vi "ELL9_Switching_with_Failed_Move_Correction.vi"() -> ()   [LabVIEW 2017]
uses:
  U:/UDocuments/Thorlabs.Elliptec.ELLO_DLL.dll
  Thorlabs.Elliptec.ELLO_DLL.dll
panel:
  in  "Stop VI":bool
  in  "COM Port":string="COM5"
  in  "Device Address":string="0"
  in  "Position 2":bool
  in  "Position 1":bool caption="Home"
  in  "Position 3":bool
  in  "Position 4":bool
  in  "Home":bool
  # "Notes:"
  # "This VI is only designed for use with the ELL9 stages.They can be running \"Daisy-Chained\" or through the ELLB Control Bus Distributor \nThe stages can not share the same address\n\nIf, when running the VI for the first time, you get a popup as illustrated below, then click Browse and navigate to the \nThorlabs.Elliptec.ELLO_DLL.dll file in the ELLO software installation directory. This can be copied to the folder you are \nrunning the VI from."
  # "Thorlabs Hardware: ELL9 - Four-Position Slider: SM1 Threads, 30 mm Cage Compatible\nhttps://www.thorlabs.com/thorproduct.cfm?partnumber=ELL9\n\nDescription: This VI will enable you to communicate with two ELL9 filter mounts. It covers connecting to the relevant COM port and addressing the desired device as well as homing the device and moving between the 16  filter positions using a case structure and while loop. \n\nIt is assumed  that you know the device address of your stage. By default this will be 0 unless changed by a user. It can be any value in Hex from 0 to F. If the device address is unknown then this is most easily found through the ELLO software: \nhttps://www.thorlabs.com/software_pages/ViewSoftwarePage.cfm?Code=ELL"
  # "Instructions:"
  # "1) Connect your devices to the USB Interface board via the ribbon cable. \n2) Connect power to the board and wait for approximately 15 seconds. As soon as the stage has power it will attempt a frequency search.\n     If the power is insufficient the board will not find the correct operating frequencies. This is why the USB is attached last. Ensure   \n     sufficient current is supplied for the number of attached stages.\n3) Connect the interface board to the PC via the USB cable.\n4) Enter the addresses of the stage you are using and the COM port you are communicating with the USB over.\n5) Run the VI.\n6) Select the position you want and allow the move to complete before choosing another."
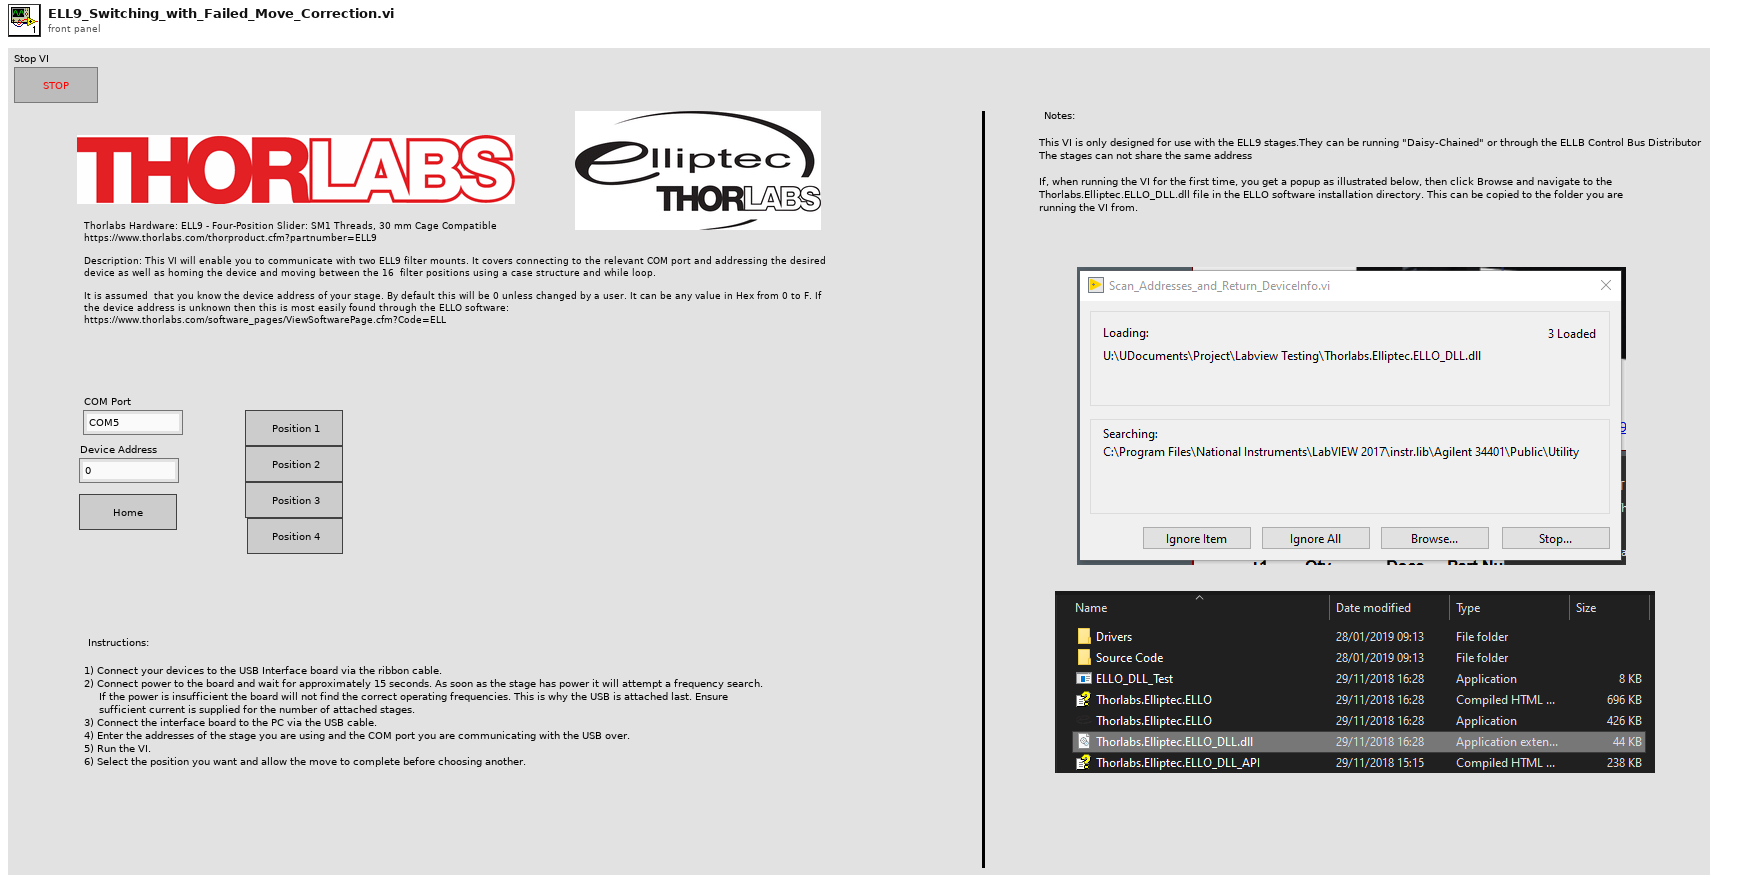
[diagram p1: front panel]
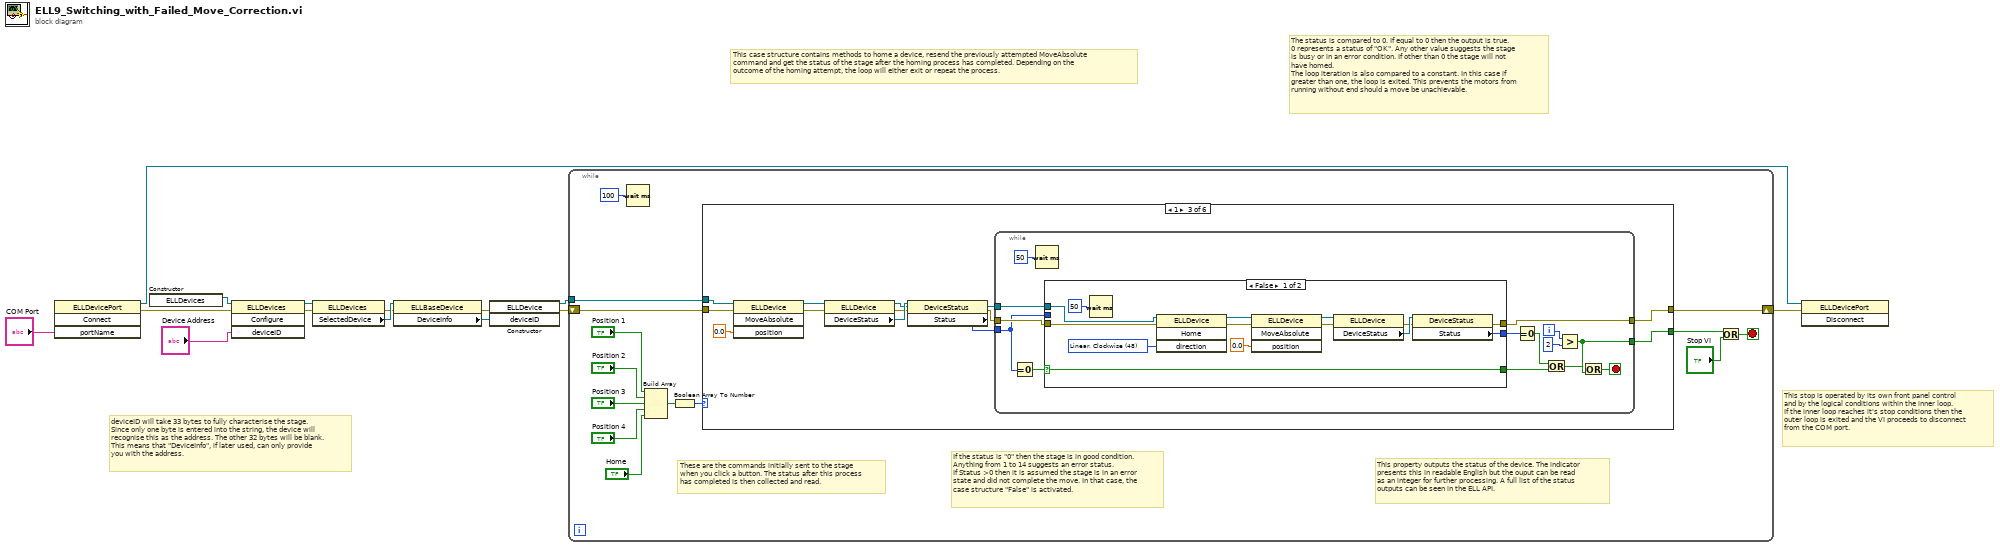
[diagram p0: block diagram]
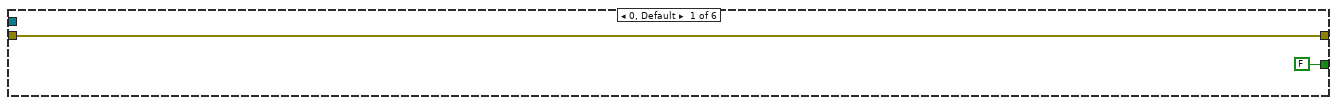
[diagram p2: hidden frame]
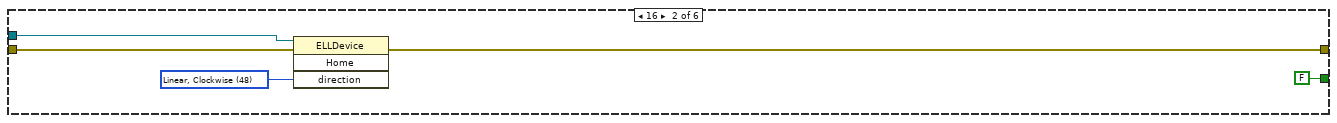
[diagram p3: hidden frame]
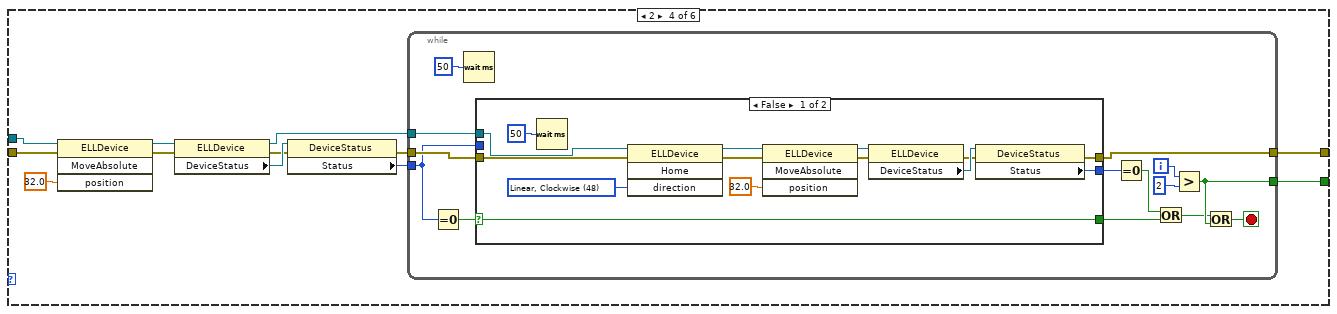
[diagram p5: hidden frame]
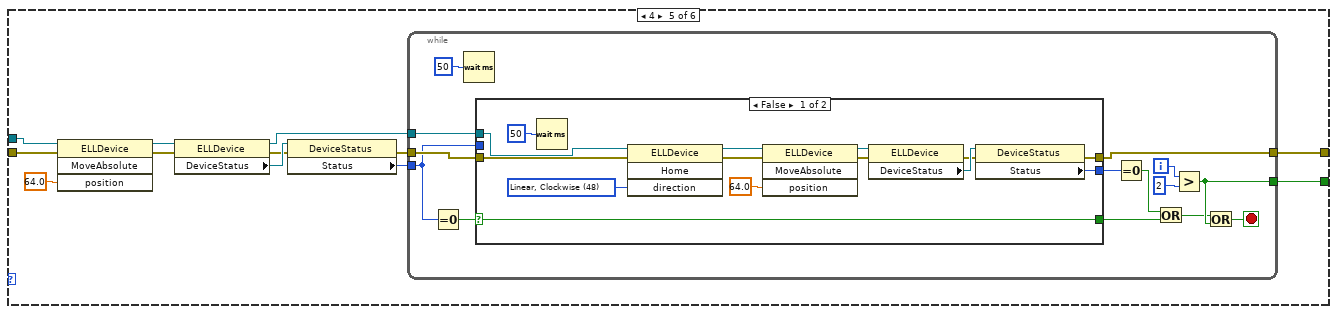
[diagram p7: hidden frame]
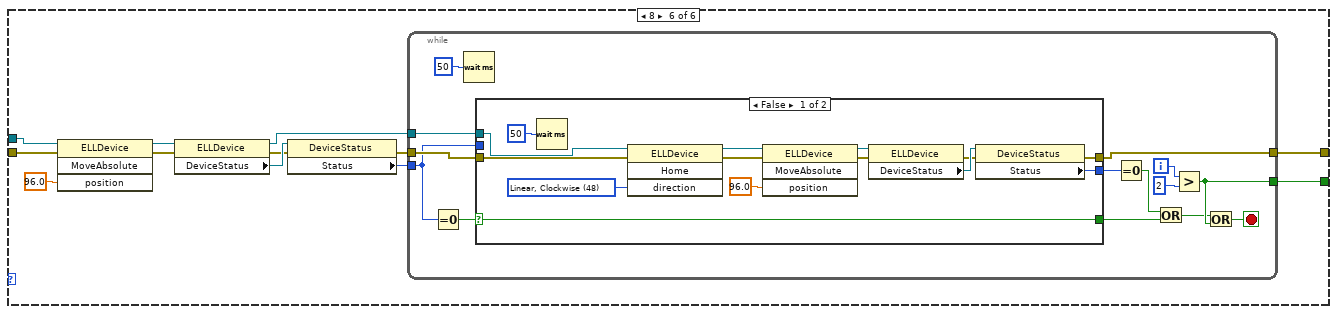
[diagram p9: hidden frame]
diagram:
  # "This case structure contains methods to home a device, resend the previously attempted MoveAbsolute \ncommand and get the status of the stage after the homing process has completed. Depending on the \noutcome of the homing attempt, the loop will either exit or repeat the process."
  # "This stop is operated by its own front panel control\nand by the logical conditions within the inner loop.\nIf the inner loop reaches it's stop conditions then the\nouter loop is exited and the VI proceeds to disconnect\nfrom the COM port."
  # "The status is compared to 0. If equal to 0 then the output is true.\n0 represents a status of \"OK\". Any other value suggests the stage\nis busy or in an error condition. If other than 0 the stage will not\nhave homed.\nThe loop iteration is also compared to a constant. In this case if\ngreater than one, the loop is exited. This prevents the motors from\nrunning without end should a move be unachievable."
  # "deviceID will take 33 bytes to fully characterise the stage. \nSince only one byte is entered into the string, the device will \nrecognise this as the address. The other 32 bytes will be blank.\nThis means that \"DeviceInfo\", if later used, can only provide \nyou with the address."
  n1 = invoke class="ELLDevicePort" method="Connect"("portName"="COM Port") -> (reference out=w14:refnum<k24>, error out=w2:errorcluster)  [unwired: 3 in, 2 out]
  n2 = constructor class="ELLDevices"() -> (reference out=w3:refnum<k24>)  [unwired: 3 in, 2 out]
  n3 = invoke class="ELLDevices" method="Configure"(reference=w3, error in=w2, "deviceID"="Device Address") -> (reference out=w11:refnum<k24>, error out=w10:errorcluster)  [unwired: 1 in, 2 out]
  n4 = property class="ELLDevices"(reference=w11, error in=w10) -> (error out=w6:errorcluster, "SelectedDevice"=w7:refnum<k24>)  [unwired: 1 out]
  n5 = property class="ELLBaseDevice"(reference=w7, error in=w6) -> (error out=w8:errorcluster, "DeviceInfo"=w9:refnum<k24>)  [unwired: 1 out]
  n6 = constructor class="ELLDevice"(error in=w8, "deviceID"=w9) -> (reference out=w5:refnum<k24>, error out=w4:errorcluster)  [unwired: 2 in, 2 out]
  n7 = while {
    shift-right: [w15] -> w13
    shift-left: w4 -> [w21]
    tunnel: w5 -> [w19]
    stop <- w18 stop-if-true
    # "These are the commands initially sent to the stage\nwhen you click a button. The status after this process\nhas completed is then collected and read."
    # "This property outputs the status of the device. The indicator\npresents this in readable English but the ouput can be read\nas an integer for further processing. A full list of the status \noutputs can be seen in the ELL API."
    # "If the status is \"0\" then the stage is in good condition.\nAnything from 1 to 14 suggests an error status. \nIf Status >0 then it is assumed the stage is in an error \nstate and did not complete the move. In that case, the\ncase structure \"False\" is activated."
    n8 = Wait (ms)(milliseconds to wait=u32 100) -> ()  [unwired: 1 out]
    n9 = Build Array("Position 1", "Position 2", "Position 3", "Position 4", "Home") -> (w28:bool[])
    n10 = Boolean Array To Number(Boolean array=w28) -> (number=w24:u32)
    n11 = case shown="1" w24 {
      tunnel: w21 -> [w30 w34 w46 w89 w132 w175]
      tunnel: w19 -> [_ w33 w45 w88 w131 w174]
      tunnel: [w30 w32 w40 w83 w126 w169] -> w15
      tunnel: [FALSE FALSE w36 w79 w122 w165] -> w17
      frame 0, Default {
      }
      frame 16 {
        w35 = 48 items=["Linear, Clockwise"=48, "AntiClockwise"=49] ("direction")
        n12 = invoke class="ELLDevice" method="Home"(reference=w33, error in=w34, "direction"=w35) -> (error out=w32:errorcluster)  [unwired: 1 in, 3 out]
      }
      frame 1 {
        n13 = invoke class="ELLDevice" method="MoveAbsolute"(reference=w45, error in=w46, "position"=0.0) -> (reference out=w42:refnum<k24>, error out=w41:errorcluster)  [unwired: 1 in, 2 out]
        n14 = property class="ELLDevice"(reference=w42, error in=w41) -> (reference out=w37:refnum<k24>, error out=w43:errorcluster, "DeviceStatus"=w44:refnum<k24>)
        n15 = property class="DeviceStatus"(reference=w44, error in=w43) -> (error out=w39:errorcluster, "Status"=w38:i32)  [unwired: 1 out]
        n16 = while {
          tunnel: [w58] -> w36
          tunnel: w37 -> [w51]
          tunnel: w38 -> [w48]
          tunnel: w39 -> [w49]
          tunnel: [w50] -> w40
          i -> [w61]
          stop <- w59 stop-if-true
          n17 = Equal To 0?(x=w48) -> (x = 0?=w53:bool)
          n18 = Wait (ms)(milliseconds to wait=u32 50) -> ()  [unwired: 1 out]
          n19 = case shown="False" w53 {
            selector: w53 -> [w62 w78]
            tunnel: w49 -> [w65 w77]
            tunnel: [w71 w76] -> w57
            tunnel: [w62 w78] -> w54
            tunnel: w51 -> [w67 _]
            tunnel: [w66 w77] -> w50
            tunnel: w48 -> [_ w76]
            frame False {
              w72 = 48 items=["Linear, Clockwise"=48, "AntiClockwise"=49] ("direction")
              n20 = Wait (ms)(milliseconds to wait=u32 50) -> ()  [unwired: 1 out]
              n21 = invoke class="ELLDevice" method="Home"(reference=w67, error in=w65, "direction"=w72) -> (reference out=w73:refnum<k24>, error out=w74:errorcluster)  [unwired: 1 in, 2 out]
              n22 = invoke class="ELLDevice" method="MoveAbsolute"(reference=w73, error in=w74, "position"=0.0) -> (reference out=w64:refnum<k24>, error out=w63:errorcluster)  [unwired: 1 in, 2 out]
              n23 = property class="ELLDevice"(reference=w64, error in=w63) -> (error out=w69:errorcluster, "DeviceStatus"=w70:refnum<k24>)  [unwired: 1 out]
              n24 = property class="DeviceStatus"(reference=w70, error in=w69) -> (error out=w66:errorcluster, "Status"=w71:i32)  [unwired: 1 out]
            }
            frame True {
            }
          }
          n25 = Equal To 0?(x=w57) -> (x = 0?=w55:bool)
          n26 = Or(x=w55, y=w54) -> (x .or. y?=w56:bool)
          n27 = Greater?(x=w61, y=2) -> (0:w58:bool)
          n28 = Or(x=w56, y=w58) -> (x .or. y?=w59:bool)
        }
      }
      frame 2 {
        n29 = invoke class="ELLDevice" method="MoveAbsolute"(reference=w88, error in=w89, "position"=32.0) -> (reference out=w85:refnum<k24>, error out=w84:errorcluster)  [unwired: 1 in, 2 out]
        n30 = property class="ELLDevice"(reference=w85, error in=w84) -> (reference out=w80:refnum<k24>, error out=w86:errorcluster, "DeviceStatus"=w87:refnum<k24>)
        n31 = property class="DeviceStatus"(reference=w87, error in=w86) -> (error out=w82:errorcluster, "Status"=w81:i32)  [unwired: 1 out]
        n32 = while {
          tunnel: [w101] -> w79
          tunnel: w80 -> [w94]
          tunnel: w81 -> [w91]
          tunnel: w82 -> [w92]
          tunnel: [w93] -> w83
          i -> [w104]
          stop <- w102 stop-if-true
          n33 = Equal To 0?(x=w91) -> (x = 0?=w96:bool)
          n34 = Wait (ms)(milliseconds to wait=u32 50) -> ()  [unwired: 1 out]
          n35 = case shown="False" w96 {
            selector: w96 -> [w105 w121]
            tunnel: w92 -> [w108 w120]
            tunnel: [w114 w119] -> w100
            tunnel: [w105 w121] -> w97
            tunnel: w94 -> [w110 _]
            tunnel: [w109 w120] -> w93
            tunnel: w91 -> [_ w119]
            frame False {
              w115 = 48 items=["Linear, Clockwise"=48, "AntiClockwise"=49] ("direction")
              n36 = Wait (ms)(milliseconds to wait=u32 50) -> ()  [unwired: 1 out]
              n37 = invoke class="ELLDevice" method="Home"(reference=w110, error in=w108, "direction"=w115) -> (reference out=w116:refnum<k24>, error out=w117:errorcluster)  [unwired: 1 in, 2 out]
              n38 = invoke class="ELLDevice" method="MoveAbsolute"(reference=w116, error in=w117, "position"=32.0) -> (reference out=w107:refnum<k24>, error out=w106:errorcluster)  [unwired: 1 in, 2 out]
              n39 = property class="ELLDevice"(reference=w107, error in=w106) -> (error out=w112:errorcluster, "DeviceStatus"=w113:refnum<k24>)  [unwired: 1 out]
              n40 = property class="DeviceStatus"(reference=w113, error in=w112) -> (error out=w109:errorcluster, "Status"=w114:i32)  [unwired: 1 out]
            }
            frame True {
            }
          }
          n41 = Equal To 0?(x=w100) -> (x = 0?=w98:bool)
          n42 = Or(x=w98, y=w97) -> (x .or. y?=w99:bool)
          n43 = Greater?(x=w104, y=2) -> (0:w101:bool)
          n44 = Or(x=w99, y=w101) -> (x .or. y?=w102:bool)
        }
      }
      frame 4 {
        n45 = invoke class="ELLDevice" method="MoveAbsolute"(reference=w131, error in=w132, "position"=64.0) -> (reference out=w128:refnum<k24>, error out=w127:errorcluster)  [unwired: 1 in, 2 out]
        n46 = property class="ELLDevice"(reference=w128, error in=w127) -> (reference out=w123:refnum<k24>, error out=w129:errorcluster, "DeviceStatus"=w130:refnum<k24>)
        n47 = property class="DeviceStatus"(reference=w130, error in=w129) -> (error out=w125:errorcluster, "Status"=w124:i32)  [unwired: 1 out]
        n48 = while {
          tunnel: [w144] -> w122
          tunnel: w123 -> [w137]
          tunnel: w124 -> [w134]
          tunnel: w125 -> [w135]
          tunnel: [w136] -> w126
          i -> [w147]
          stop <- w145 stop-if-true
          n49 = Equal To 0?(x=w134) -> (x = 0?=w139:bool)
          n50 = Wait (ms)(milliseconds to wait=u32 50) -> ()  [unwired: 1 out]
          n51 = case shown="False" w139 {
            selector: w139 -> [w148 w164]
            tunnel: w135 -> [w151 w163]
            tunnel: [w157 w162] -> w143
            tunnel: [w148 w164] -> w140
            tunnel: w137 -> [w153 _]
            tunnel: [w152 w163] -> w136
            tunnel: w134 -> [_ w162]
            frame False {
              w158 = 48 items=["Linear, Clockwise"=48, "AntiClockwise"=49] ("direction")
              n52 = Wait (ms)(milliseconds to wait=u32 50) -> ()  [unwired: 1 out]
              n53 = invoke class="ELLDevice" method="Home"(reference=w153, error in=w151, "direction"=w158) -> (reference out=w159:refnum<k24>, error out=w160:errorcluster)  [unwired: 1 in, 2 out]
              n54 = invoke class="ELLDevice" method="MoveAbsolute"(reference=w159, error in=w160, "position"=64.0) -> (reference out=w150:refnum<k24>, error out=w149:errorcluster)  [unwired: 1 in, 2 out]
              n55 = property class="ELLDevice"(reference=w150, error in=w149) -> (error out=w155:errorcluster, "DeviceStatus"=w156:refnum<k24>)  [unwired: 1 out]
              n56 = property class="DeviceStatus"(reference=w156, error in=w155) -> (error out=w152:errorcluster, "Status"=w157:i32)  [unwired: 1 out]
            }
            frame True {
            }
          }
          n57 = Equal To 0?(x=w143) -> (x = 0?=w141:bool)
          n58 = Or(x=w141, y=w140) -> (x .or. y?=w142:bool)
          n59 = Greater?(x=w147, y=2) -> (0:w144:bool)
          n60 = Or(x=w142, y=w144) -> (x .or. y?=w145:bool)
        }
      }
      frame 8 {
        n61 = invoke class="ELLDevice" method="MoveAbsolute"(reference=w174, error in=w175, "position"=96.0) -> (reference out=w171:refnum<k24>, error out=w170:errorcluster)  [unwired: 1 in, 2 out]
        n62 = property class="ELLDevice"(reference=w171, error in=w170) -> (reference out=w166:refnum<k24>, error out=w172:errorcluster, "DeviceStatus"=w173:refnum<k24>)
        n63 = property class="DeviceStatus"(reference=w173, error in=w172) -> (error out=w168:errorcluster, "Status"=w167:i32)  [unwired: 1 out]
        n64 = while {
          tunnel: [w187] -> w165
          tunnel: w166 -> [w180]
          tunnel: w167 -> [w177]
          tunnel: w168 -> [w178]
          tunnel: [w179] -> w169
          i -> [w190]
          stop <- w188 stop-if-true
          n65 = Equal To 0?(x=w177) -> (x = 0?=w182:bool)
          n66 = Wait (ms)(milliseconds to wait=u32 50) -> ()  [unwired: 1 out]
          n67 = case shown="False" w182 {
            selector: w182 -> [w191 w207]
            tunnel: w178 -> [w194 w206]
            tunnel: [w200 w205] -> w186
            tunnel: [w191 w207] -> w183
            tunnel: w180 -> [w196 _]
            tunnel: [w195 w206] -> w179
            tunnel: w177 -> [_ w205]
            frame False {
              w201 = 48 items=["Linear, Clockwise"=48, "AntiClockwise"=49] ("direction")
              n68 = Wait (ms)(milliseconds to wait=u32 50) -> ()  [unwired: 1 out]
              n69 = invoke class="ELLDevice" method="Home"(reference=w196, error in=w194, "direction"=w201) -> (reference out=w202:refnum<k24>, error out=w203:errorcluster)  [unwired: 1 in, 2 out]
              n70 = invoke class="ELLDevice" method="MoveAbsolute"(reference=w202, error in=w203, "position"=96.0) -> (reference out=w193:refnum<k24>, error out=w192:errorcluster)  [unwired: 1 in, 2 out]
              n71 = property class="ELLDevice"(reference=w193, error in=w192) -> (error out=w198:errorcluster, "DeviceStatus"=w199:refnum<k24>)  [unwired: 1 out]
              n72 = property class="DeviceStatus"(reference=w199, error in=w198) -> (error out=w195:errorcluster, "Status"=w200:i32)  [unwired: 1 out]
            }
            frame True {
            }
          }
          n73 = Equal To 0?(x=w186) -> (x = 0?=w184:bool)
          n74 = Or(x=w184, y=w183) -> (x .or. y?=w185:bool)
          n75 = Greater?(x=w190, y=2) -> (0:w187:bool)
          n76 = Or(x=w185, y=w187) -> (x .or. y?=w188:bool)
        }
      }
    }
    n77 = Or(x=w17, y="Stop VI") -> (x .or. y?=w18:bool)
  }
  n78 = invoke class="ELLDevicePort" method="Disconnect"(reference=w14, error in=w13) -> ()  [unwired: 1 in, 3 out]
